vi "newChipKick.vi"(0 "Game":refnum<class "Game.lvclass">, 2 "Target":dbl[](array[numeric]), 3 "use criteria?":bool, 5 "shootState?":bool, 6 "pass ?":bool, 7 "Robot":refnum<class "Robot.lvclass">, 9 "Robot Pos":dbl[](array[numeric]), 13 "chipKick ?":bool) -> (4 "ChipKick Force":dbl)   [LabVIEW 2023, in "KickToSkill.lvclass"]
uses:
  KickToSkill.lvclass
  Game_class/Game.lvclass
  Robot_class/Robot.lvclass
  C:/Users/lucio/Desktop/roboime/SSL_AI/Object_class/Object.lvclass
  Team_class/KeeperPlay.ctl
  Game_class/Game.lvclass/Game.ctl
  Team_class/Team.lvclass/Team.ctl
  Parameters_class/Parameters.lvclass/Parameters.ctl
  Referee_class/Referee.lvclass/Referee.ctl
  Robot_class/Robot.lvclass/Robot.ctl
  Object_class/Object.lvclass/Object.ctl
  Robot_class/roles.ctl
  Utilities_class/Utilities.lvclass
  Parameters_class/Read ChipKick Force 1.vi
  Object_class/Read x.vi
  Object_class/Read y.vi
  Robot_class/Read id.vi
  Robot_class/Read role.vi
  Game_class/Read KeeperTeam.vi
  Game_class/Read Parameters.lvclass.vi
  Game_class/Read EnemyRef.vi
  Game_class/Read BallRef.vi
  Game_class/Read FieldRef.vi
  Game_class/Read Referee.vi
  Referee_class/Read our_goalie_id.vi
  Parameters_class/Read ChipKick activated.vi
  Team_class/Read KeeperPlay.vi
  Ally_class/Ally.lvclass
  C:/Users/lucio/Desktop/roboime/SSL_AI/Team_class/Team.lvclass
  Ball_class/Ball.lvclass
  Parameters_class/Parameters.lvclass
  Enemy_class/Enemy.lvclass
  Field_class/Field.lvclass
  Referee_class/Referee.lvclass
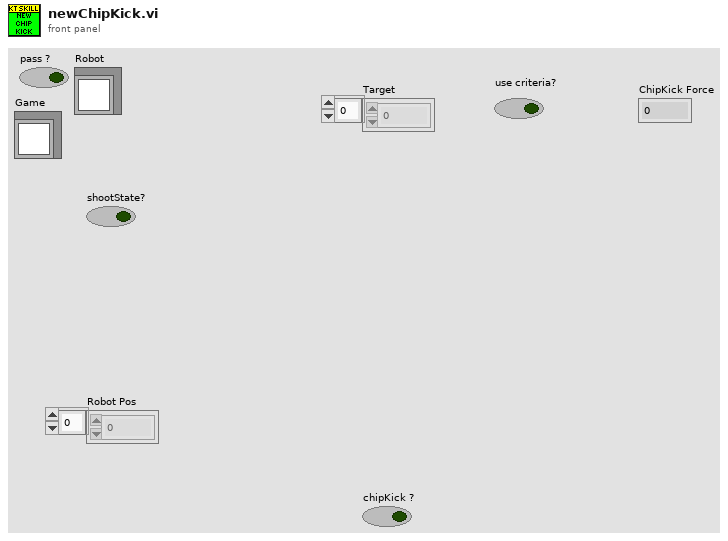
[diagram p1: front panel]
types:
  T1 = typedef "KeeperPlay.ctl" = enum16{"SimpleBallPlacementAlly", "BallPlacementAlly", "BallPlacementEnemy", "ZigZag", "Goto", "NormalGame", "KeeperPlay", "Halt", "Timeout", "PenaltyEnemy", "TestPlay"}
  T2 = typedef "roles.ctl" = enum16{"SimpleBallPlacement", "BallPlacementAllyPasser", "BallPlacementAllyReceiver", "BallPlacementEnemy", "5Robots5th", "PassBestReceiver", "5Robots4th", "5Robots3rd", "5Robots2nd", "5Robots1st", "PassBestRobot", "WaitPass", "ABCThirdKicker", "ABCFirstKicker", "ABCSecondKicker", "Tabler", "TableFinalizer", "PrepareRollToPassRoller", "PrepareRollToPassReceiver", "SimplePassRoll", "SimplePassRollReceiver", "PenaltyDefense", "PreparePassReceiver 2", "PreparePassReceiver 1", "PassObserver", "Timeout", "Goto", "ZigZag", "None", "BallOutOfField", "DefenderArea", "Duelist", "AttackerStop", "FollowAttacker", "KeeperRole", "KickPenalty", "AttackerAimGoal", "AttackerBlock", "Marker", "Halt", "Shoot", "PassKicker", "PassReceiver", "TestRole", "PenaltyAttacker"}
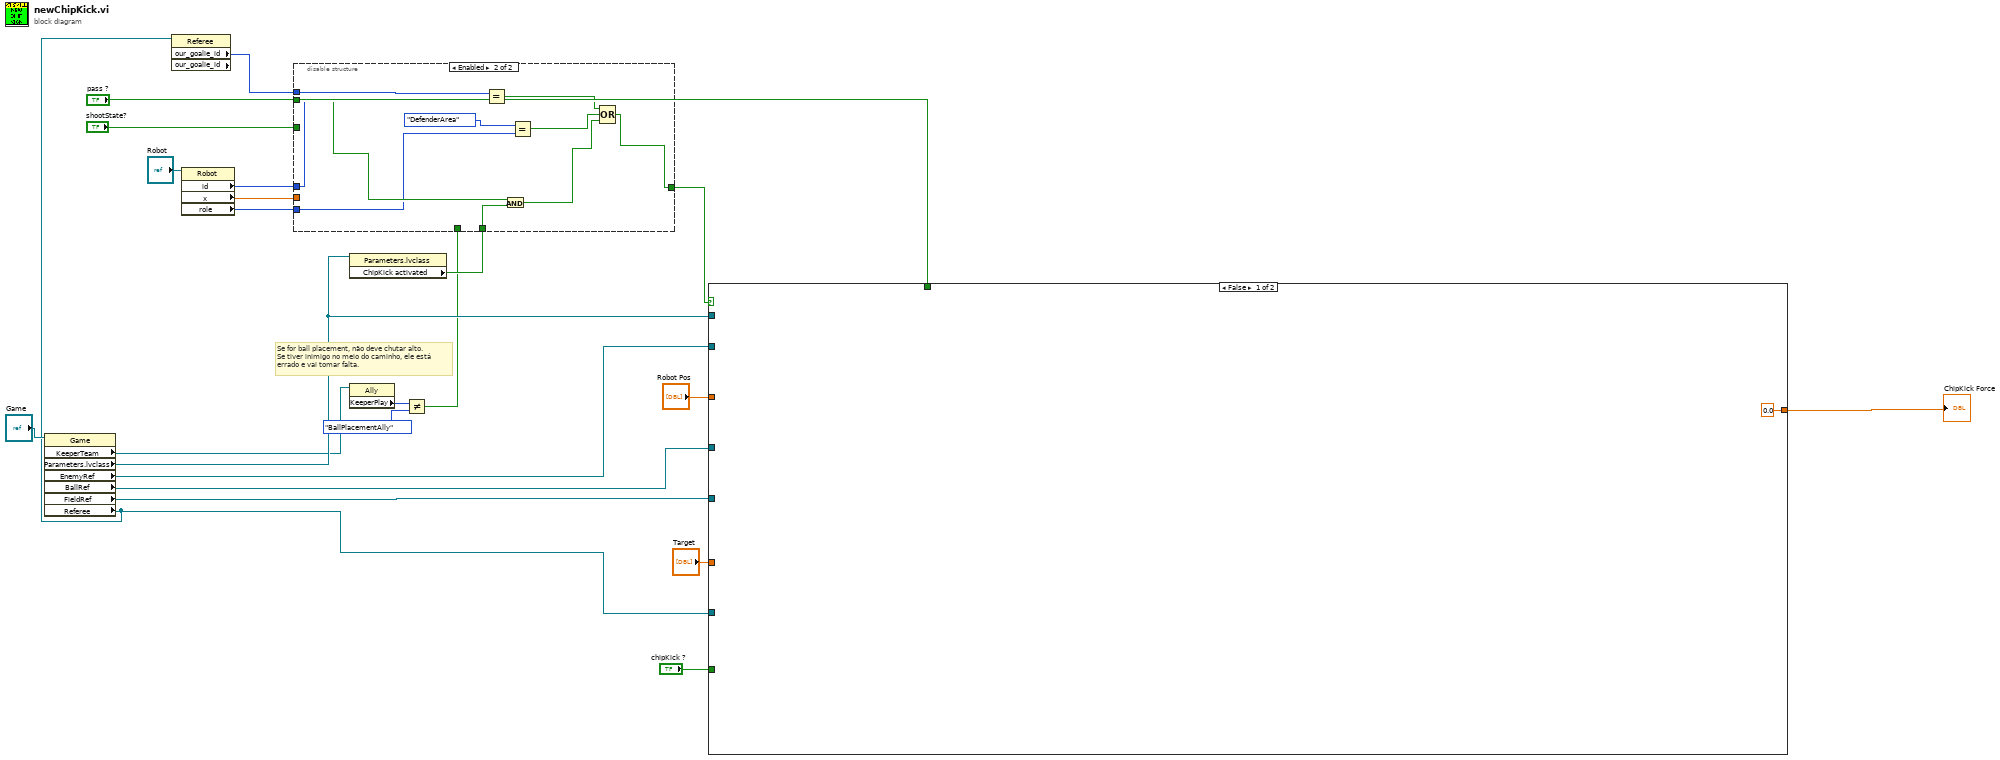
[diagram p0: block diagram]
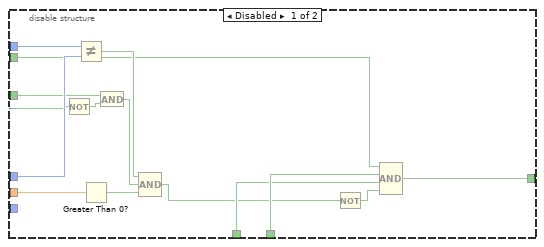
[diagram p2: hidden frame]
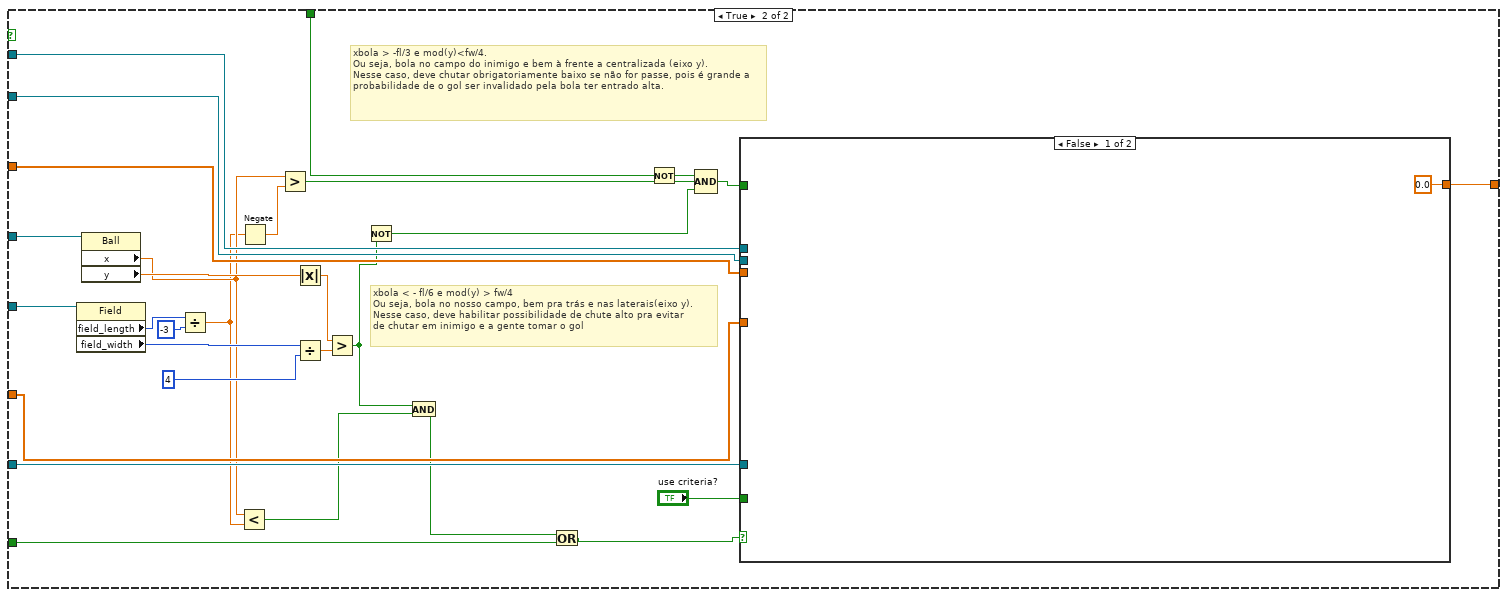
[diagram p3: hidden frame]
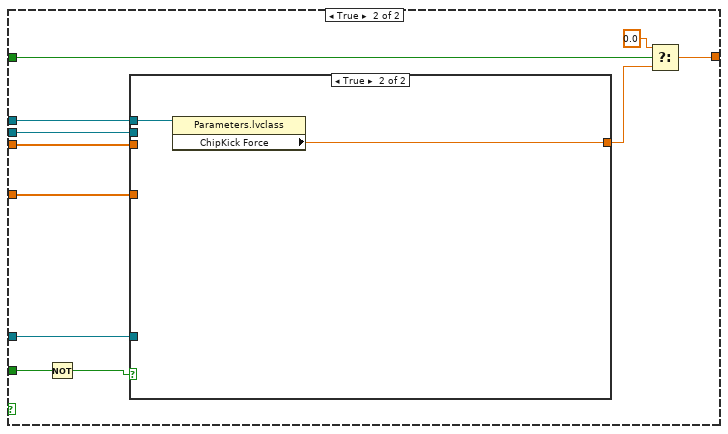
[diagram p4: hidden frame]
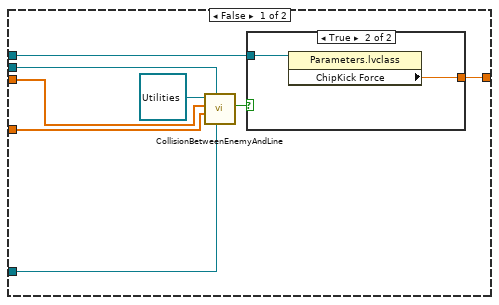
[diagram p5: hidden frame]
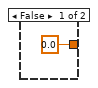
[diagram p6: hidden frame]
diagram:
  # "Se for ball placement, não deve chutar alto.\nSe tiver inimigo no meio do caminho, ele está\nerrado e vai tomar falta."
  n1 = property class="Game"(reference="Game") -> ("KeeperTeam"=w13:refnum<class "Ally.lvclass">, "Parameters.lvclass"=w14:refnum<class "Parameters.lvclass">, "EnemyRef"=w16:refnum<class "Enemy.lvclass">, "BallRef"=w15:refnum<class "Ball.lvclass">, "FieldRef"=w5:refnum<class "Field.lvclass">, "Referee"=w6:refnum<class "Referee.lvclass">)  [unwired: 1 in, 2 out]
  n2 = property class="Referee" props=["our_goalie_id", "our_goalie_id"](reference=w6) -> ("our_goalie_id"=w8:i32)  [unwired: 1 in, 3 out]
  n3 = property class="Robot"(reference="Robot") -> ("id"=w7:i32, "x"=w4:dbl, "role"=w1:T2)  [unwired: 1 in, 2 out]
  n4 = property class="Ally"(reference=w13) -> ("KeeperPlay"=w12:T1)  [unwired: 1 in, 2 out]
  n5 = property class="Parameters.lvclass"(reference=w14) -> ("ChipKick activated"=w18:bool)  [unwired: 1 in, 2 out]
  n6 = Not Equal?(x=w12, y=KeeperPlay."BallPlacementAlly") -> (x != y?=w10:bool)
  n7 = disable-structure shown="Enabled" {
    disable-tunnel: [w37 w40] -> w19
    disable-tunnel: w18 -> [w36 w45]
    disable-tunnel: w10 -> [w35 _]
    disable-tunnel: w8 -> [w33 w47]
    disable-tunnel: w7 -> [w32 w46]
    disable-tunnel: w4 -> [w27 _]
    disable-tunnel: "shootState?" -> [w26 _]
    disable-tunnel: "pass ?" -> [w24 w44]
    disable-tunnel: w1 -> [_ w43]
    frame Disabled {
      n8 = Not(x=w24) -> (.not. x?=w28:bool)
      n9 = Not Equal?(x=w33, y=w32) -> (x != y?=w31:bool)
      n10 = Greater Than 0?(x=w27) -> (x > 0?=w29:bool)
      n11 = And(x=w26, y=w28) -> (x .and. y?=w25:bool)
      n12 = Compound Arithmetic op=AND(w31, w25, w29) -> (w30:bool)
      n13 = Not(x=w30) -> (.not. x?=w34:bool)
      n14 = Compound Arithmetic op=AND(w24, w36, w35, w34) -> (w37:bool)
    }
    frame Enabled {
      n15 = Equal?(x=w47, y=w46) -> (x = y?=w38:bool)
      n16 = And(x=w44, y=w45) -> (x .and. y?=w41:bool)
      n17 = Equal?(x=roles."DefenderArea" ("role"), y=w43) -> (x = y?=w39:bool)
      n18 = Compound Arithmetic op=OR(w38, w39, w41) -> (w40:bool)
    }
  }
  n19 = case shown="False" w19 {
    tunnel: [0.0 ("ChipKick Force") w77] -> w22
    tunnel: "Robot Pos" -> [_ w75]
    tunnel: "Target" -> [_ w74]
    tunnel: w14 -> [_ w73]
    tunnel: "chipKick ?" -> [_ w51]
    tunnel: w16 -> [_ w72]
    tunnel: w15 -> [_ w71]
    tunnel: w5 -> [_ w70]
    tunnel: w6 -> [_ w62]
    tunnel: "pass ?" -> [_ w50]
    frame False {
    }
    frame True {
      # "xbola > -fl/3 e mod(y)<fw/4.\nOu seja, bola no campo do inimigo e bem à frente a centralizada (eixo y).\nNesse caso, deve chutar obrigatoriamente baixo se não for passe, pois é grande a probabilidade de o gol ser invalidado pela bola ter entrado alta."
      # "xbola < - fl/6 e mod(y) > fw/4\nOu seja, bola no nosso campo, bem pra trás e nas laterais(eixo y).\nNesse caso, deve habilitar possibilidade de chute alto pra evitar\nde chutar em inimigo e a gente tomar o gol"
      n20 = property class="Field"(reference=w70) -> ("field_length"=w69:i32, "field_width"=w65:i32)  [unwired: 1 in, 2 out]
      n21 = property class="Ball"(reference=w71) -> ("x"=w61:dbl, "y"=w67:dbl)  [unwired: 1 in, 2 out]
      n22 = Divide(x=w69, y=-3) -> (x/y=w60:dbl)
      n23 = Less?(x=w61, y=w60) -> (x < y?=w53:bool)
      n24 = Negate(x=w60) -> (-x=w56:dbl)
      n25 = Greater?(x=w61, y=w56) -> (0:w59:bool)
      n26 = Absolute Value(x=w67) -> (abs(x)=w66:dbl)
      n27 = Divide(x=w65, y=4) -> (x/y=w63:dbl)
      n28 = Greater?(x=w66, y=w63) -> (0:w54:bool)
      n29 = Not(x=w54) -> (.not. x?=w57:bool)
      n30 = And(x=w54, y=w53) -> (x .and. y?=w52:bool)
      n31 = Or(x=w52, y=w51) -> (x .or. y?=w49:bool)
      n32 = Not(x=w50) -> (.not. x?=w55:bool)
      n33 = Compound Arithmetic op=AND(w55, w59, w57) -> (w58:bool)
      n34 = case shown="False" w49 {
        tunnel: [0.0 w80] -> w77
        tunnel: "use criteria?" -> [_ w85]
        tunnel: w73 -> [_ w89]
        tunnel: w75 -> [_ w88]
        tunnel: w74 -> [_ w87]
        tunnel: w72 -> [_ w86]
        tunnel: w62 -> [_ w84]
        tunnel: w58 -> [_ w82]
        frame False {
        }
        frame True {
          n35 = Not(x=w85) -> (.not. x?=w79:bool)
          n36 = case shown="True" w79 {
            tunnel: w89 -> [w92 w102]
            tunnel: [w93 w101] -> w83
            tunnel: w88 -> [w96 _]
            tunnel: w87 -> [w95 _]
            tunnel: w86 -> [w91 _]
            tunnel: w84 -> [w90 _]
            frame False {
              n37 = call-dynamic "CollisionBetweenEnemyAndLine.vi"("Referee"=w90, "EnemyRef"=w91, "P2"=w95, "P1"=w96, "Utilities in"=refnum<class "Utilities.lvclass"> refnum) -> ("collision ?"=w94:bool)  [unwired: 3 in, 3 out]
              n38 = case shown="True" w94 {
                tunnel: [0.0 w100] -> w93
                tunnel: w92 -> [_ w99]
                frame False {
                }
                frame True {
                  n39 = property class="Parameters.lvclass"(reference=w99) -> ("ChipKick Force"=w100:dbl)  [unwired: 1 in, 2 out]
                }
              }
            }
            frame True {
              n40 = property class="Parameters.lvclass"(reference=w102) -> ("ChipKick Force"=w101:dbl)  [unwired: 1 in, 2 out]
            }
          }
          n41 = Select(t=0.0, s=w82, f=w83) -> (s? t:f=w80:dbl)
        }
      }
    }
  }
  "ChipKick Force" <- w22
